vi "Fetch Waveform.vi"(8 "error in (no error)":errorcluster, 10 "Channel":u8, 11 "Scope PXI Base CFG in":refnum<class "Scope PXI Base CFG.lvclass">) -> (0 "error out":errorcluster, 2 "Waveform":waveform(dbl), 3 "Scope PXI Base CFG out":refnum<class "Scope PXI Base CFG.lvclass">)   [LabVIEW 2023, in "Scope PXI Base CFG.lvclass"]
uses:
  Scope PXI Base CFG.lvclass
  <instrlib>/niScope/Controls/niScope timestamp type.ctl
  Scope PXI Base CFG.lvclass/Scope PXI Base CFG.ctl
  Configuration/Configuration JSON/Configuration JSON Base/CFG JSON.lvclass/CFG JSON.ctl
  9a7c277c-3744-422f-a2d5-5dbb7f71351f.vi
  <vilib>/JDP Science/JSONtext/Find Item.vi
  <vilib>/JDP Science/JSONtext/Next JSON Value.vi
  <vilib>/JDP Science/JSONtext/String Subset.vi
  <vilib>/JDP Science/JSONtext/Parsing/Advance past next JSON Value (inlined COPY).vi
  <vilib>/JDP Science/JSONtext/Parsing/Advance past whitespace.vi
  <vilib>/JDP Science/JSONtext/Parsing/Advance past String.vi
  <vilib>/JDP Science/JSONtext/Parsing/Advance past Number.vi
  <vilib>/JDP Science/JSONtext/Parsing/Advance past Line Ending.vi
  <vilib>/JDP Science/JSONtext/Parsing/Parse Full Path or Item Name.vi
  <vilib>/JDP Science/JSONtext/Parsing/Advance past Array.vi
  <vilib>/JDP Science/JSONtext/Parsing/Advance past Object.vi
  <vilib>/JDP Science/JSONtext/support/Error Cluster From Code.vi
  <vilib>/JDP Science/JSONtext/Offset/Find Item Locations by Path.vi
  <vilib>/JDP Science/JSONtext/JSON text to Variant.vi
  <vilib>/Utility/error.llb/Error Cluster From Error Code.vi
  <instrlib>/niScope/Acquire/Fetch/niScope Fetch WDT.vi
  <vilib>/JDP Science/JSONtext/LVClass Serializer/JSONtext LVClass Serializer.lvclass
  <vilib>/ErrorRing/Error Ring.xnode
  Configuration/Configuration JSON/Configuration JSON Base/CFG JSON.lvclass
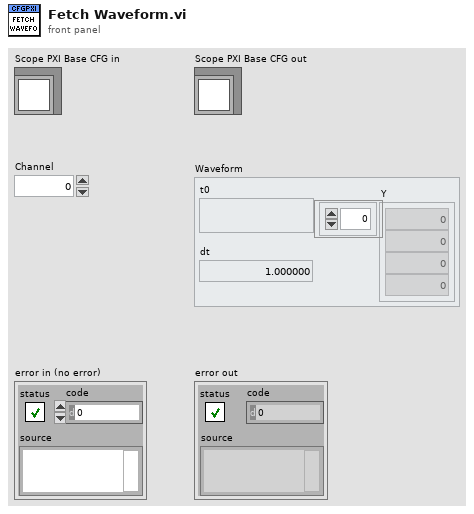
[diagram p1: front panel]
types:
  T1 = typedef "niScope timestamp type.ctl" = i32
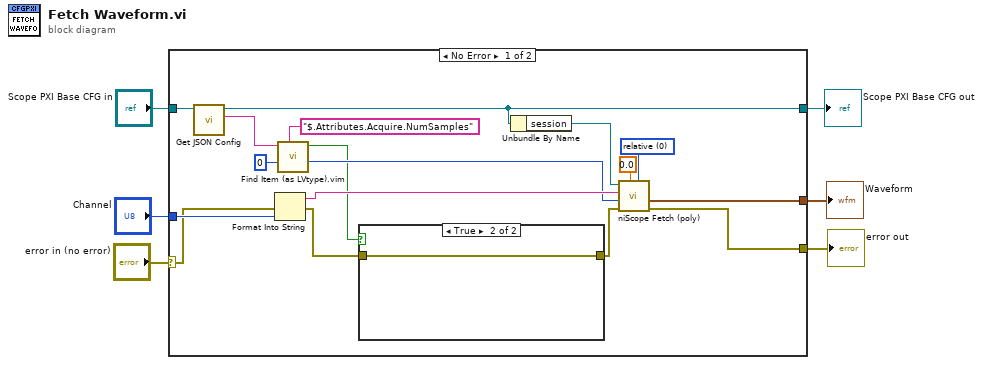
[diagram p0: block diagram]
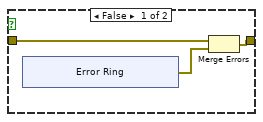
[diagram p2: hidden frame]
diagram:
  n1 = case shown="No Error" "error in (no error)" {
    selector: "error in (no error)" -> [w7 w34]
    tunnel: [w23 w34] -> w5
    tunnel: [w15 w33] -> w3
    tunnel: "Scope PXI Base CFG in" -> [w22 w33]
    tunnel: "Channel" -> [w18 _]
    tunnel: [w16 _] -> w1
    frame No Error {
      w8 = T1 0 items=["relative", "absolute"] ("timestamp Type")
      n2 = call "Get JSON Config.vi"("CFG Base in"=w22) -> ("<JSON>Config>"=w19:string, "CFG Base out"=w15:refnum<class "Scope PXI Base CFG.lvclass">)  [unwired: 9 in]
      n3 = Format Into String(error in=w7, w18) -> (resulting string=w17:string, error out=w12:errorcluster)  [unwired: 2 in]
      n4 = call "Find Item (as LVtype).vim"("$Path or Item Name"="$.Attributes.Acquire.NumSamples", "Data Type and Default Value"=0, "JSON"=w19) -> ("Data"=w13:i32, "Found"=w10:bool)  [unwired: 5 in, 2 out]
      n5 = case shown="True" w10 {
        tunnel: w12 -> [w26 w32]
        tunnel: [w25 w32] -> w11
        frame False {
          n6 = xnode "Error Ring"() -> ("error out"=w24:errorcluster)
          n7 = Merge Errors(w26, w24) -> (w25:errorcluster)
        }
        frame True {
        }
      }
      n8 = Unbundle By Name(w15) -> ("session"=w14:refnum<k15>)
      n9 = call-poly <instrlib>:"niScope Fetch (poly).vi"("timestamp Type"=w8, "timeout"=0.0, "error in"=w11, "numSamples"=w13, "channels"=w17, "instrument handle"=w14) -> ("error out"=w23:errorcluster, "wfm"=w16:waveform(dbl))  [unwired: 2 in, 2 out]
    }
    frame Error {
    }
  }
  "error out" <- w5
  "Scope PXI Base CFG out" <- w3
  "Waveform" <- w1
